vi "GEOM_GetDETNFO.vi"(8 "error in (no error)":errorcluster, 10 "detnum":u16) -> (0 "error out":errorcluster, 2 "info":string)   [LabVIEW 2016]
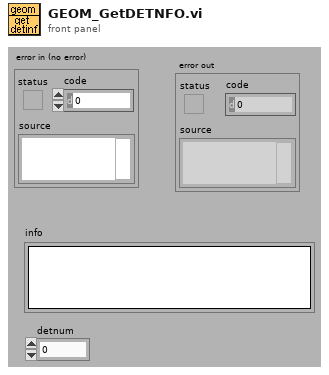
[diagram p1: front panel]
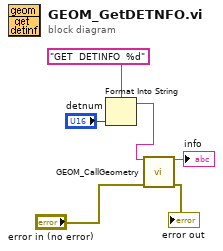
[diagram p0: block diagram]
diagram:
  n1 = Format Into String(format string="GET  DETINFO  %d" ("string (\"\")"), "detnum") -> (resulting string=w2:string)  [unwired: 2 in, 1 out]
  n2 = call "GEOM_CallGeometry.vi"("Command"=w2, "error in (no error)"="error in (no error)") -> ("ImmedReplyString"=→"info":string, "error out"=→"error out":errorcluster)  [unwired: 12 out]
